vi "Update.vi"(8 "error in (no error)":errorcluster, 10 "Model in":refnum<class "Model.lvclass">, 11 "Perform Open Loop Scan State in":refnum<class "Perform Open Loop Scan State.lvclass">) -> (0 "error out":errorcluster, 2 "Model out":refnum<class "Model.lvclass">, 3 "Perform Open Loop Scan State out":refnum<class "Perform Open Loop Scan State.lvclass">)   [LabVIEW 2015, in "Perform Open Loop Scan State.lvclass"]
uses:
  Perform Open Loop Scan State.lvclass
  Model/Model/Model.lvclass
  Typedefs/State Types.ctl
  Typedefs/FAMT Typedefs.lvlib
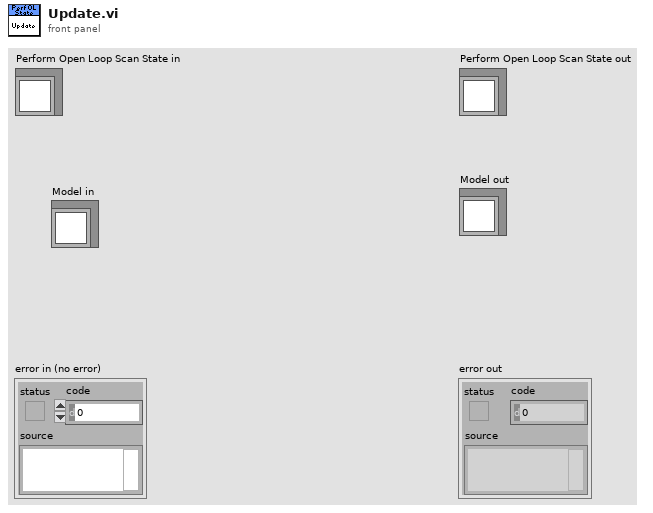
[diagram p1: front panel]
types:
  T1 = typedef "FAMT Typedefs.lvlib/State Types.ctl" = enum16{"Offline State", "Fault State", "Standby State", "Disabled State", "Enabled State", "Wait For User Input State", "Perform Open Loop Scan State", "Perform Closed Loop Scan State"}
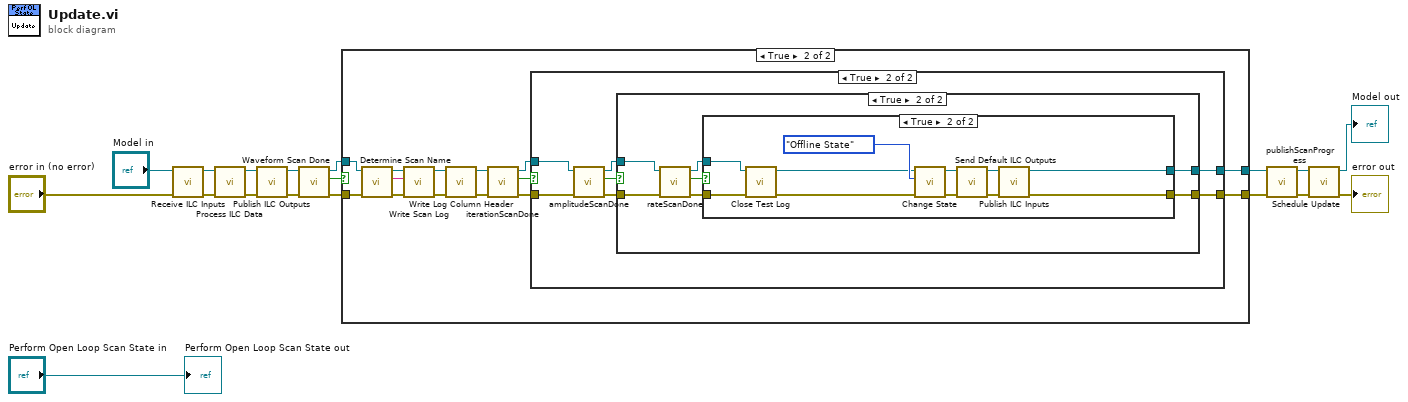
[diagram p0: block diagram]
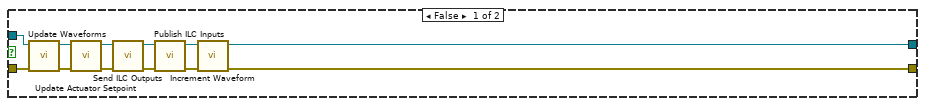
[diagram p2: hidden frame]
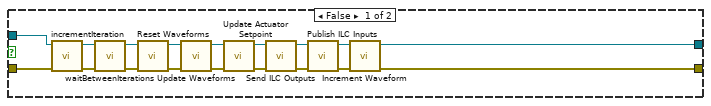
[diagram p3: hidden frame]
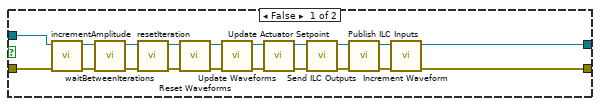
[diagram p4: hidden frame]
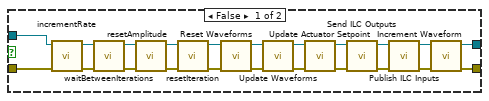
[diagram p5: hidden frame]
diagram:
  n1 = call "Receive ILC Inputs.vi"("error in (no error)"="error in (no error)", "Model in"="Model in") -> ("error out"=w1:errorcluster, "Model out"=w2:refnum<class "Model.lvclass">)  [unwired: 8 in]
  n2 = call "Process ILC Data.vi"("error in (no error)"=w1, "Model in"=w2) -> ("error out"=w9:errorcluster, "Model out"=w18:refnum<class "Model.lvclass">)  [unwired: 8 in]
  n3 = call "Publish ILC Outputs.vi"("error in (no error)"=w9, "Model in"=w18) -> ("error out"=w8:errorcluster, "Model out"=w12:refnum<class "Model.lvclass">)  [unwired: 8 in]
  n4 = call "Waveform Scan Done.vi"("error in (no error)"=w8, "Model in"=w12) -> ("error out"=w7:errorcluster, "Done"=w14:bool, "Model out"=w13:refnum<class "Model.lvclass">)  [unwired: 7 in]
  n5 = case shown="True" w14 {
    tunnel: w13 -> [w25 w38]
    tunnel: [w19 w31] -> w6
    tunnel: [w27 w44] -> w11
    tunnel: w7 -> [w24 w36]
    frame False {
      n6 = call "Update Waveforms.vi"("error in (no error)"=w24, "Model in"=w25) -> ("error out"=w23:errorcluster, "Model out"=w26:refnum<class "Model.lvclass">)  [unwired: 8 in]
      n7 = call "Update Actuator Setpoint.vi"("error in (no error)"=w23, "Model in"=w26) -> ("error out"=w22:errorcluster, "Model out"=w30:refnum<class "Model.lvclass">)  [unwired: 8 in]
      n8 = call "Send ILC Outputs.vi"("error in (no error)"=w22, "Model in"=w30) -> ("error out"=w21:errorcluster, "Model out"=w29:refnum<class "Model.lvclass">)  [unwired: 8 in]
      n9 = call "Publish ILC Inputs.vi"("error in (no error)"=w21, "Model in"=w29) -> ("error out"=w20:errorcluster, "Model out"=w28:refnum<class "Model.lvclass">)  [unwired: 8 in]
      n10 = call "Increment Waveform.vi"("error in (no error)"=w20, "Model in"=w28) -> ("error out"=w19:errorcluster, "Model out"=w27:refnum<class "Model.lvclass">)  [unwired: 8 in]
    }
    frame True {
      n11 = call "Determine Scan Name.vi"("error in (no error)"=w36, "Model in"=w38) -> ("error out"=w35:errorcluster, "Scan Name"=w37:string, "Model out"=w39:refnum<class "Model.lvclass">)  [unwired: 7 in]
      n12 = call "Write Scan Log.vi"("error in (no error)"=w35, "File Name"=w37, "Model in"=w39) -> ("error out"=w34:errorcluster, "Model out"=w41:refnum<class "Model.lvclass">)  [unwired: 7 in]
      n13 = call "Write Log Column Header.vi"("error in (no error)"=w34, "Model in"=w41) -> ("error out"=w33:errorcluster, "Model out"=w40:refnum<class "Model.lvclass">)  [unwired: 8 in]
      n14 = call "iterationScanDone.vi"("error in (no error)"=w33, "Model in"=w40) -> ("error out"=w32:errorcluster, "Done?"=w43:bool, "Model out"=w42:refnum<class "Model.lvclass">)  [unwired: 7 in]
      n15 = case shown="True" w43 {
        tunnel: w42 -> [w56 w67]
        tunnel: [w45 w63] -> w31
        tunnel: [w57 w66] -> w44
        tunnel: w32 -> [w53 w65]
        frame False {
          n16 = call "incrementIteration.vi"("error in (no error)"=w53, "Model in"=w56) -> ("error out"=w52:errorcluster, "Model out"=w55:refnum<class "Model.lvclass">)  [unwired: 8 in]
          n17 = call "waitBetweenIterations.vi"("error in (no error)"=w52, "Model in"=w55) -> ("error out"=w51:errorcluster, "Model out"=w54:refnum<class "Model.lvclass">)  [unwired: 8 in]
          n18 = call "Reset Waveforms.vi"("error in (no error)"=w51, "Model in"=w54) -> ("error out"=w50:errorcluster, "Model out"=w58:refnum<class "Model.lvclass">)  [unwired: 8 in]
          n19 = call "Update Waveforms.vi"("error in (no error)"=w50, "Model in"=w58) -> ("error out"=w49:errorcluster, "Model out"=w59:refnum<class "Model.lvclass">)  [unwired: 8 in]
          n20 = call "Update Actuator Setpoint.vi"("error in (no error)"=w49, "Model in"=w59) -> ("error out"=w48:errorcluster, "Model out"=w62:refnum<class "Model.lvclass">)  [unwired: 8 in]
          n21 = call "Send ILC Outputs.vi"("error in (no error)"=w48, "Model in"=w62) -> ("error out"=w47:errorcluster, "Model out"=w61:refnum<class "Model.lvclass">)  [unwired: 8 in]
          n22 = call "Publish ILC Inputs.vi"("error in (no error)"=w47, "Model in"=w61) -> ("error out"=w46:errorcluster, "Model out"=w60:refnum<class "Model.lvclass">)  [unwired: 8 in]
          n23 = call "Increment Waveform.vi"("error in (no error)"=w46, "Model in"=w60) -> ("error out"=w45:errorcluster, "Model out"=w57:refnum<class "Model.lvclass">)  [unwired: 8 in]
        }
        frame True {
          n24 = call "amplitudeScanDone.vi"("error in (no error)"=w65, "Model in"=w67) -> ("error out"=w64:errorcluster, "Done?"=w69:bool, "Model out"=w68:refnum<class "Model.lvclass">)  [unwired: 7 in]
          n25 = case shown="True" w69 {
            tunnel: w68 -> [w89 w95]
            tunnel: [w70 w90] -> w63
            tunnel: [w85 w93] -> w66
            tunnel: w64 -> [w79 w92]
            frame False {
              n26 = call "incrementAmplitude.vi"("error in (no error)"=w79, "Model in"=w89) -> ("error out"=w78:errorcluster, "Model out"=w81:refnum<class "Model.lvclass">)  [unwired: 8 in]
              n27 = call "waitBetweenIterations.vi"("error in (no error)"=w78, "Model in"=w81) -> ("error out"=w77:errorcluster, "Model out"=w80:refnum<class "Model.lvclass">)  [unwired: 8 in]
              n28 = call "resetIteration.vi"("error in (no error)"=w77, "Model in"=w80) -> ("error out"=w76:errorcluster, "Model out"=w82:refnum<class "Model.lvclass">)  [unwired: 8 in]
              n29 = call "Reset Waveforms.vi"("error in (no error)"=w76, "Model in"=w82) -> ("error out"=w75:errorcluster, "Model out"=w84:refnum<class "Model.lvclass">)  [unwired: 8 in]
              n30 = call "Update Waveforms.vi"("error in (no error)"=w75, "Model in"=w84) -> ("error out"=w74:errorcluster, "Model out"=w83:refnum<class "Model.lvclass">)  [unwired: 8 in]
              n31 = call "Update Actuator Setpoint.vi"("error in (no error)"=w74, "Model in"=w83) -> ("error out"=w73:errorcluster, "Model out"=w88:refnum<class "Model.lvclass">)  [unwired: 8 in]
              n32 = call "Send ILC Outputs.vi"("error in (no error)"=w73, "Model in"=w88) -> ("error out"=w72:errorcluster, "Model out"=w87:refnum<class "Model.lvclass">)  [unwired: 8 in]
              n33 = call "Publish ILC Inputs.vi"("error in (no error)"=w72, "Model in"=w87) -> ("error out"=w71:errorcluster, "Model out"=w86:refnum<class "Model.lvclass">)  [unwired: 8 in]
              n34 = call "Increment Waveform.vi"("error in (no error)"=w71, "Model in"=w86) -> ("error out"=w70:errorcluster, "Model out"=w85:refnum<class "Model.lvclass">)  [unwired: 8 in]
            }
            frame True {
              n35 = call "rateScanDone.vi"("error in (no error)"=w92, "Model in"=w95) -> ("error out"=w91:errorcluster, "Done?"=w96:bool, "Model out"=w94:refnum<class "Model.lvclass">)  [unwired: 7 in]
              n36 = case shown="True" w96 {
                tunnel: w94 -> [w115 w125]
                tunnel: [w97 w119] -> w90
                tunnel: [w114 w126] -> w93
                tunnel: w91 -> [w107 w123]
                frame False {
                  n37 = call "incrementRate.vi"("error in (no error)"=w107, "Model in"=w115) -> ("error out"=w106:errorcluster, "Model out"=w109:refnum<class "Model.lvclass">)  [unwired: 8 in]
                  n38 = call "waitBetweenIterations.vi"("error in (no error)"=w106, "Model in"=w109) -> ("error out"=w105:errorcluster, "Model out"=w108:refnum<class "Model.lvclass">)  [unwired: 8 in]
                  n39 = call "resetAmplitude.vi"("error in (no error)"=w105, "Model in"=w108) -> ("error out"=w104:errorcluster, "Model out"=w111:refnum<class "Model.lvclass">)  [unwired: 8 in]
                  n40 = call "resetIteration.vi"("error in (no error)"=w104, "Model in"=w111) -> ("error out"=w103:errorcluster, "Model out"=w110:refnum<class "Model.lvclass">)  [unwired: 8 in]
                  n41 = call "Reset Waveforms.vi"("error in (no error)"=w103, "Model in"=w110) -> ("error out"=w102:errorcluster, "Model out"=w113:refnum<class "Model.lvclass">)  [unwired: 8 in]
                  n42 = call "Update Waveforms.vi"("error in (no error)"=w102, "Model in"=w113) -> ("error out"=w101:errorcluster, "Model out"=w112:refnum<class "Model.lvclass">)  [unwired: 8 in]
                  n43 = call "Update Actuator Setpoint.vi"("error in (no error)"=w101, "Model in"=w112) -> ("error out"=w100:errorcluster, "Model out"=w118:refnum<class "Model.lvclass">)  [unwired: 8 in]
                  n44 = call "Send ILC Outputs.vi"("error in (no error)"=w100, "Model in"=w118) -> ("error out"=w99:errorcluster, "Model out"=w117:refnum<class "Model.lvclass">)  [unwired: 8 in]
                  n45 = call "Publish ILC Inputs.vi"("error in (no error)"=w99, "Model in"=w117) -> ("error out"=w98:errorcluster, "Model out"=w116:refnum<class "Model.lvclass">)  [unwired: 8 in]
                  n46 = call "Increment Waveform.vi"("error in (no error)"=w98, "Model in"=w116) -> ("error out"=w97:errorcluster, "Model out"=w114:refnum<class "Model.lvclass">)  [unwired: 8 in]
                }
                frame True {
                  n47 = call "Close Test Log.vi"("error in (no error)"=w123, "Model in"=w125) -> ("error out"=w122:errorcluster, "Model out"=w124:refnum<class "Model.lvclass">)  [unwired: 8 in]
                  n48 = call "Change State.vi"("error in (no error)"=w122, "State Types"=State_Types."Offline State" ("State:"), "Model in"=w124) -> ("error out"=w121:errorcluster, "Model out"=w128:refnum<class "Model.lvclass">)  [unwired: 7 in]
                  n49 = call "Send Default ILC Outputs.vi"("error in (no error)"=w121, "Model in"=w128) -> ("error out"=w120:errorcluster, "Model out"=w127:refnum<class "Model.lvclass">)  [unwired: 8 in]
                  n50 = call "Publish ILC Inputs.vi"("error in (no error)"=w120, "Model in"=w127) -> ("error out"=w119:errorcluster, "Model out"=w126:refnum<class "Model.lvclass">)  [unwired: 8 in]
                }
              }
            }
          }
        }
      }
    }
  }
  n51 = call "publishScanProgress.vi"("error in (no error)"=w6, "Model in"=w11) -> ("error out"=w5:errorcluster, "Model out"=w15:refnum<class "Model.lvclass">)  [unwired: 8 in]
  n52 = call "Schedule Update.vi"("error in (no error)"=w5, "Model in"=w15) -> ("error out"=→"error out":errorcluster, "Model out"=→"Model out":refnum<class "Model.lvclass">)  [unwired: 8 in]
  "Perform Open Loop Scan State out" <- "Perform Open Loop Scan State in"
